vi "_Read Voltage.vi"(0 "LINX Resource in":T1, 2 "Single-Diff Select (Diff)":enum16{"Differential", "Single-Ended"}(ring), 3 "Channel Select (CH0)":T9(ring), 5 "error in (no error)":errorcluster, 8 "CS Configuration":T7={"CS Channel"=7, "CS Logic Level"=enum."Active Low"}, 9 "Vref (3.3V)":dbl=3.3, 10 "SPI Channel (0)":u8) -> (13 "L":u8 format="%.0x", 14 "LINX Resource out":T1, 16 "Converted Voltage (V)":dbl, 17 "12-bit ADC Code":u16 format="%.0x", 18 "H":u8 format="%.0x", 19 "error out":errorcluster)   [LabVIEW 2014]
doc: "<b>-------------------------------------------------------</b>\n** Author: Derek Murray\n** Created: 08/08/2016\n** LV Version: LabVIEW 2014 Home SP1 (14.0.1f3 32-bit)\n<b>-------------------------------------------------------</b>\n\nReads the voltage on a particular channel of the MCP3008 ADC. Vref is the reference voltage for ADC conversions and is the voltage applied to pin 15 of the MCP3008. If 'Single-Diff Select' is set to single-ended, then the common ground for voltage conversions is AGND (pin 14), and the positive voltage is connected to CH0 to CH7. The 'Channel Select' control allows the channel to be set. If the mode is differential, then the channel connections are shown in brackets in the 'Channel Select' enum. They are:\n\nD2 D1 D0\n0 0 0 => CH0 = IN+, CH1 = IN-\n0 0 1 => CH1 = IN+, CH0 = IN-\n0 1 0 => CH2 = IN+, CH3 = IN-\n0 1 1 => CH3 = IN+, CH2 = IN-\n1 0 0 => CH4 = IN+, CH5 = IN-\n1 0 1 => CH5 = IN+, CH4 = IN-\n1 1 0 => CH6 = IN+, CH7 = IN-\n1 1 1 => CH7 = IN+, CH6 = IN-\n\n<b>-------------------------------------------------------</b>\n** Copyright/License\nPermission is hereby granted, free of charge, to any person obtaining a copy of this software and associated documentation files (the \"Software\"), to deal in the Software without restriction, including without limitation the rights to use, copy, modify, merge, publish, distribute, sublicense, and/or sell copies of the Software, and to permit persons to whom the Software is furnished to do so, subject to the following conditions:\nThe above copyright notice and this permission notice shall be included in all copies or substantial portions of the Software.\nTHE SOFTWARE IS PROVIDED \"AS IS\", WITHOUT WARRANTY OF ANY KIND, EXPRESS OR IMPLIED, INCLUDING BUT NOT LIMITED TO THE WARRANTIES OF MERCHANTABILITY, FITNESS FOR A PARTICULAR PURPOSE AND NONINFRINGEMENT. IN NO EVENT SHALL THE AUTHORS OR COPYRIGHT HOLDERS BE LIABLE FOR ANY CLAIM, DAMAGES OR OTHER LIABILITY, WHETHER IN AN ACTION OF CONTRACT, TORT OR OTHERWISE, ARISING FROM, OUT OF OR IN CONNECTION WITH THE SOFTWARE OR THE USE OR OTHER DEALINGS IN THE SOFTWARE."
uses:
  <vilib>/MakerHub/LINX/Public/Peripherals/SPI/SPI CS Config.ctl
  <vilib>/MakerHub/LINX/Private/Type Defs/Peripherals/SPI/SPI CS Logic Level.ctl
  <vilib>/MakerHub/LINX/Private/Type Defs/LINX Ref.ctl
  <vilib>/MakerHub/LINX/Private/Type Defs/Platform.ctl
  <vilib>/MakerHub/LINX/Private/Type Defs/Interface.ctl
  <vilib>/MakerHub/LINX/Private/Device/Type Defs/LINX Device Config.ctl
  <vilib>/MakerHub/LINX/Private/Device/Type Defs/TCP Config.ctl
  <vilib>/MakerHub/LINX/Private/Device/Type Defs/Channels.ctl
  <vilib>/MakerHub/LINX/Public/Peripherals/SPI/SPI Write Read 1 Frame.vi
  <vilib>/MakerHub/LINX/Public/Peripherals/SPI/SPI Write Read N Frames.vi
  <vilib>/MakerHub/LINX/Private/Local IO/LinxSpiWriteRead.vi
  <vilib>/MakerHub/LINX/Public/Utilities/Check Channel.vi
  <vilib>/MakerHub/LINX/Private/Local IO/Handle Errors.vi
  <vilib>/MakerHub/LINX/Private/Utilties/Generate Error.vi
  <vilib>/MakerHub/LINX/LMH-LINX.lvlib
  <vilib>/MakerHub/LINX/Private/Device/Device.lvlib
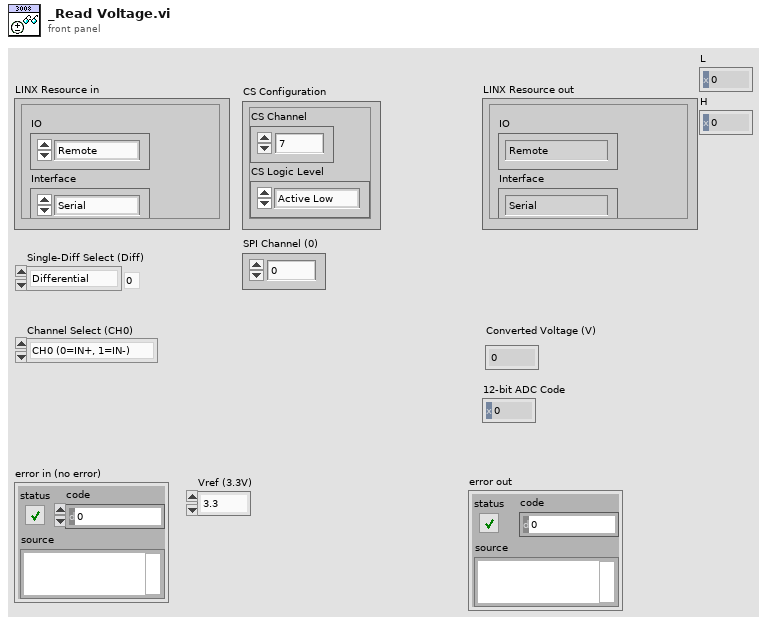
[diagram p1: front panel]
types:
  T1 = typedef "LMH-LINX.lvlib/LINX Ref.ctl" = cluster{"IO":T2, "Interface":T3, "LINX Device Config":T4}
  T2 = typedef "LMH-LINX.lvlib/Platform.ctl" = enum16{"Remote", "Local"}
  T3 = typedef "LMH-LINX.lvlib/Interface.ctl" = enum16{"Serial", "TCP"}
  T4 = typedef "LMH-LINX.lvlib/Device.lvlib/LINX Device Config.ctl" = cluster{"Interface":T3, "COM Port":refnum<visa-resource-name>, "TCP Configuration":T5, "Device Family":u8, "Device ID":u8, "Device Name":string, "TCP Ref":refnum<k5>, "Channels":T6}
  T5 = typedef "LMH-LINX.lvlib/Device.lvlib/TCP Config.ctl" = cluster{"IP Address":string, "Port":u16}
  T6 = typedef "LMH-LINX.lvlib/Channels.ctl" = cluster{"DI":u8[], "DO":u8[], "AI":u8[], "AO":u8[], "PWM":u8[], "QE":u8[], "UART":u8[], "I2C 2":u8[], "SPI":u8[], "CAN":u8[], "Servo":u8[], "AI Ref (V)":dbl, "AI Resolution (Bits)":u8, "AO Ref (V)":dbl, "AO Resolution (Bits)":u8}
  T7 = typedef "LMH-LINX.lvlib/SPI CS Config.ctl" = cluster{"CS Channel":u8, "CS Logic Level":T8}
  T8 = typedef "LMH-LINX.lvlib/SPI CS Logic Level.ctl" = enum8{"Active Low", "Active High"}
  T9 = enum16{"CH0 (0=IN+, 1=IN-)", "CH1 (1=IN+, 0=IN-)", "CH2 (2=IN+, 3=IN-)", "CH3 (3=IN+, 2=IN-)", "CH4 (4=IN+, 5=IN-)", "CH5 (5=IN+, 4=IN-)", "CH6 (6=IN+, 7=IN-)", "CH7 (7=IN+, 6=IN-)"}
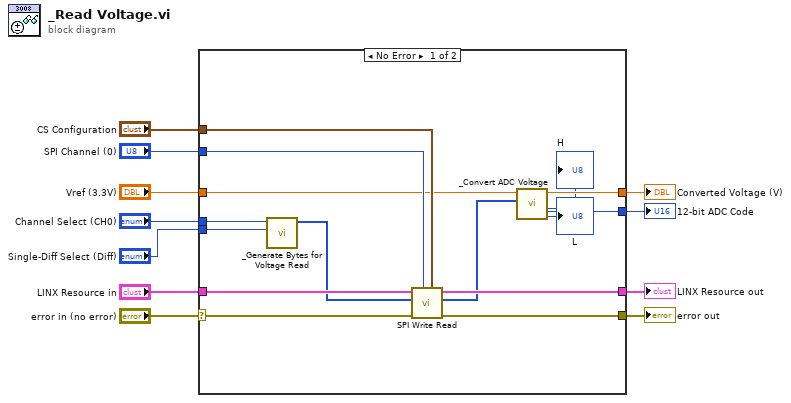
[diagram p0: block diagram]
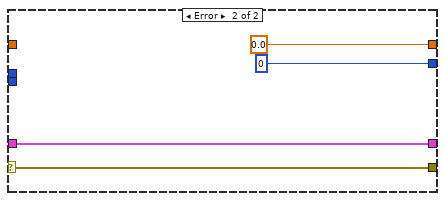
[diagram p2: hidden frame]
diagram:
  n1 = case shown="No Error" "error in (no error)" {
    selector: "error in (no error)" -> [w22 w29]
    tunnel: "CS Configuration" -> [w26 _]
    tunnel: [w25 w29] -> w10
    tunnel: [w24 w30] -> w9
    tunnel: "LINX Resource in" -> [w23 w30]
    tunnel: "SPI Channel (0)" -> [w21 _]
    tunnel: "Channel Select (CH0)" -> [w20 _]
    tunnel: "Single-Diff Select (Diff)" -> [w19 _]
    tunnel: "Vref (3.3V)" -> [w16 _]
    tunnel: [w15 0.0 ("Converted Voltage (V)")] -> w2
    tunnel: [w14 u16 0 ("10-bit ADC Code")] -> w1
    frame No Error {
      n2 = call "_Generate Bytes for Voltage Read.vi"("Single-Diff Select (Diff)"=w19, "Channel Select (CH0)"=w20) -> ("Write Data1"=w18:u8[])  [unwired: 9 in]
      n3 = call-poly <vilib>:"SPI Write Read.vi"("CS Configuration"=w26, "SPI Channel (0)"=w21, "Error In"=w22, "Data"=w18, "LINX Resource"=w23) -> ("Error Out"=w25:errorcluster, "Read Data"=w17:u8[], "LINX Resource"=w24:T1)  [unwired: 4 in]
      n4 = call "_Convert ADC Voltage.vi"("SPI Read Array"=w17, "Vref (3.3V)"=w16) -> ("L"=→"L":u8, "H"=→"H":u8, "12-bit ADC Code"=w14:u16, "Converted Voltage (V)"=w15:dbl)  [unwired: 6 in]
    }
    frame Error {
    }
  }
  "12-bit ADC Code" <- w1
  "Converted Voltage (V)" <- w2
  "error out" <- w10
  "LINX Resource out" <- w9
